vi "Select Category ID by Name.vi"(8 "error in (no error)":errorcluster, 10 "Category Name":string, 11 "Database in":refnum<class "Database.lvclass">) -> (0 "error out":errorcluster, 2 "Category ID":i32, 3 "Database out":refnum<class "Database.lvclass">)   [LabVIEW 2018, in "Database.lvclass"]
uses:
  Database.lvclass
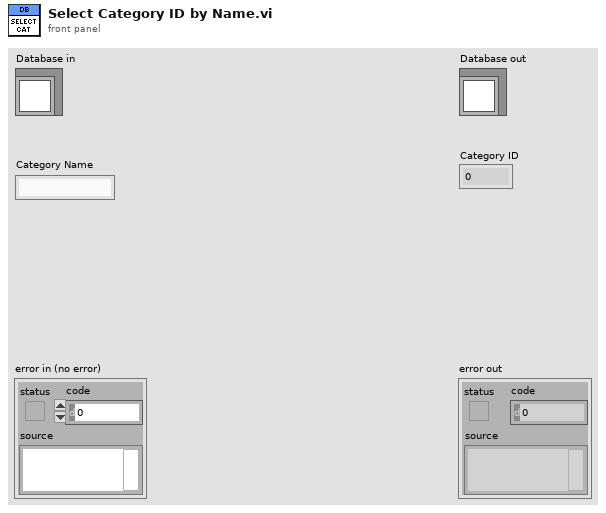
[diagram p1: front panel]
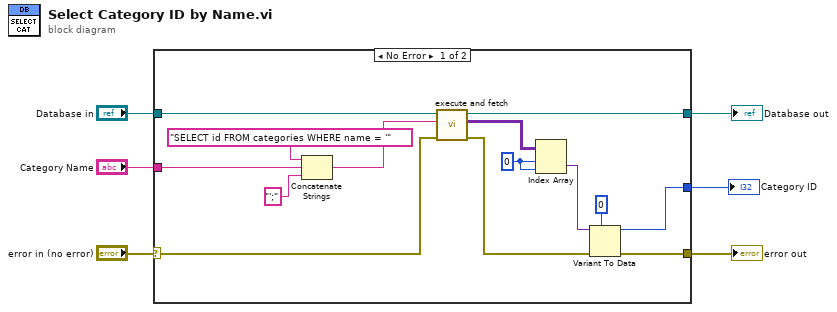
[diagram p0: block diagram]
diagram:
  n1 = case shown="No Error" "error in (no error)" {
    selector: "error in (no error)" -> [w7 w21]
    tunnel: "Database in" -> [w17 w22]
    tunnel: [w16 w22] -> w5
    tunnel: "Category Name" -> [w15 _]
    tunnel: [w9 w21] -> w3
    tunnel: [w8 _] -> w2
    frame No Error {
      w12 = 0 ("index (row)")
      n2 = Concatenate Strings("SELECT id FROM categories WHERE name = '", w15, "';") -> (w18:string)
      n3 = call "execute and fetch.vi"("error in (no error)"=w7, "SQL query"=w18, "Database in"=w17) -> ("error out"=w10:errorcluster, "recordset data"=w13:variant[][], "Database out"=w16:refnum<class "Database.lvclass">)  [unwired: 5 in, 1 out]
      n4 = Index Array(array=w13, index (row)=w12, index (col)=w12) -> (element=w11:variant)
      n5 = Variant To Data(error in=w10, type=0, Variant=w11) -> (data=w8:i32, error out=w9:errorcluster)
    }
    frame Error {
    }
  }
  "error out" <- w3
  "Database out" <- w5
  "Category ID" <- w2
